vi "MW_SweepFrequency.vi"(8 "错误输入（无错误）":errorcluster, 9 "iteration":i32, 10 "MW Source Freq.":T1, 11 "VISA引用句柄输入":refnum<visa-resource-name>) -> (0 "错误输出":errorcluster, 1 "Finished?":bool, 2 "Set Frequency":dbl, 3 "VISA引用句柄输出":refnum<visa-resource-name>, 4 "Command":string)   [LabVIEW 2016, in "Microwave Source.lvlib"]
uses:
  Microwave Source.lvlib
  MW_ctl_Souce Freq..ctl
panel:
  out "Freq":dbl
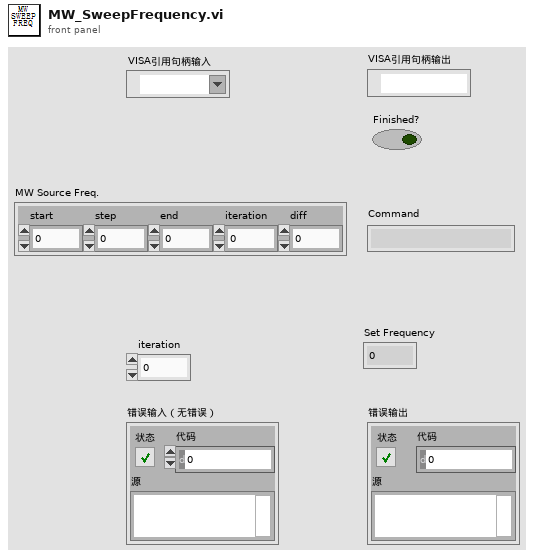
[diagram p1: front panel]
types:
  T1 = typedef "Microwave Source.lvlib/MW_ctl_Souce Freq..ctl" = cluster{"start":dbl, "step":dbl, "end":dbl, "iteration":dbl, "diff":dbl}
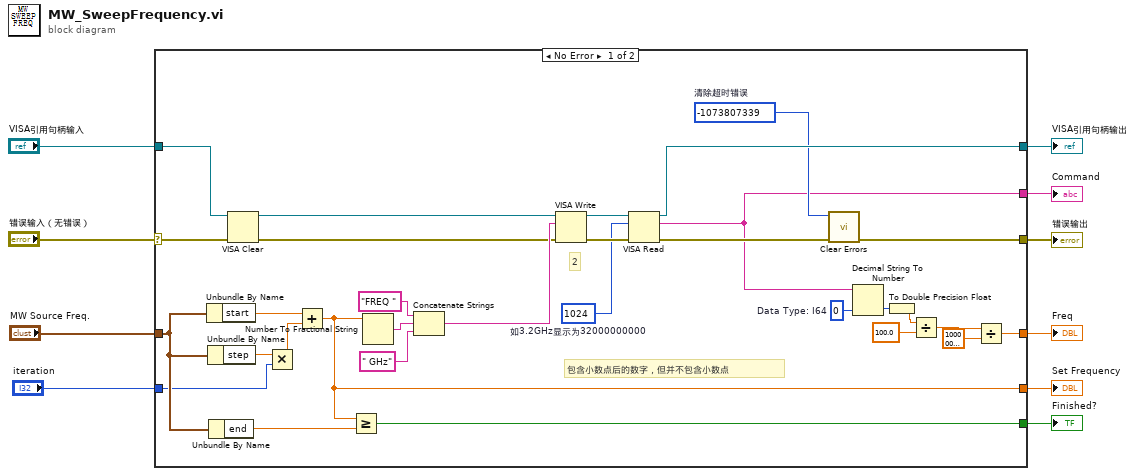
[diagram p0: block diagram]
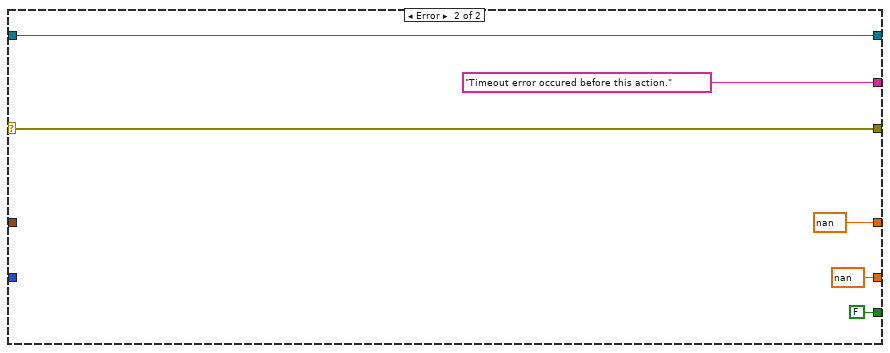
[diagram p2: hidden frame]
diagram:
  n1 = case shown="No Error" "错误输入（无错误）" {
    selector: "错误输入（无错误）" -> [w14 w47]
    tunnel: "VISA引用句柄输入" -> [w13 w46]
    tunnel: [w40 w46] -> w3
    tunnel: [w35 w47] -> w2
    tunnel: [w34 "Timeout error occured before this action." ("read buffer")] -> w4
    tunnel: [w28 nan] -> w5
    tunnel: "MW Source Freq." -> [w24 _]
    tunnel: "iteration" -> [w22 _]
    tunnel: [w18 FALSE] -> w6
    tunnel: [w16 nan] -> w1
    frame No Error {
      w33 = i64 0  # Data Type: I64
      w37 = -1073807339  # 清除超时错误
      w38 = u32 1024  # 如3.2GHz显示为32000000000
      # "包含小数点后的数字，但并不包含小数点"
      # "2"
      n2 = Unbundle By Name(w24) -> ("start"=w26:dbl)
      n3 = Unbundle By Name(w24) -> ("step"=w27:dbl)
      n4 = Unbundle By Name(w24) -> ("end"=w23:dbl)
      n5 = VISA Clear(VISA resource name=w13, error in (no error)=w14) -> (VISA resource name out=w12:refnum<visa-resource-name>, error out=w15:errorcluster)
      n6 = Multiply(x=w27, y=w22) -> (x*y=w25:dbl)
      n7 = Add(x=w26, y=w25) -> (x+y=w16:dbl)
      n8 = Greater Or Equal?(x=w16, y=w23) -> (x >= y?=w18:bool)
      n9 = Number To Fractional String(number=w16) -> (F-format string=w19:string)  [unwired: 3 in]
      n10 = Concatenate Strings("FREQ ", w19, " GHz") -> (w17:string)
      n11 = VISA Write(VISA resource name=w12, write buffer=w17, error in (no error)=w15) -> (VISA resource name out=w41:refnum<visa-resource-name>, error out=w39:errorcluster)  [unwired: 1 out]
      n12 = VISA Read(VISA resource name=w41, byte count=w38, error in (no error)=w39) -> (VISA resource name out=w40:refnum<visa-resource-name>, read buffer=w34:string, error out=w36:errorcluster)  [unwired: 1 out]
      n13 = call <vilib>:"Clear Errors.vi"("error in (no error)"=w36, "specific error code to clear (0: all)"=w37) -> ("error out"=w35:errorcluster)  [unwired: 4 in, 1 out]
      n14 = Decimal String To Number(string=w34, default (0L)=w33) -> (number=w32:i64)  [unwired: 1 in, 1 out]
      n15 = To Double Precision Float(number=w32) -> (double precision float=w11:dbl)
      n16 = Divide(x=w11, y=100.0) -> (x/y=w29:dbl)
      n17 = Divide(x=w29, y=1000000000.0) -> (x/y=w28:dbl)
    }
    frame Error {
    }
  }
  "Freq" <- w5
  "Command" <- w4
  "错误输出" <- w2
  "VISA引用句柄输出" <- w3
  "Finished?" <- w6
  "Set Frequency" <- w1
